vi "Global Aquatrak Output.vi"(0 "AT In":string, 3 "Set Data?":bool) -> (7 "AT Out":string)   [LabVIEW 2018]
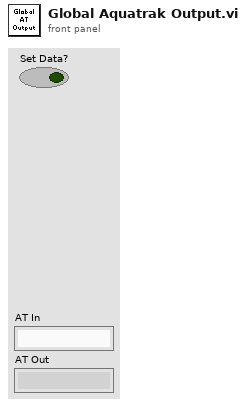
[diagram p1: front panel]
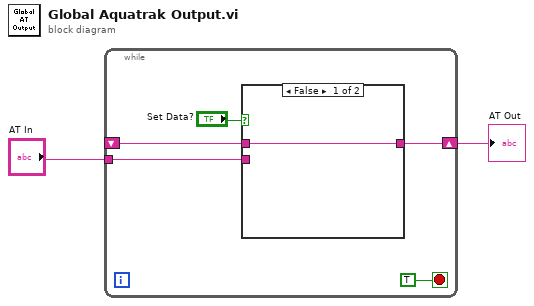
[diagram p0: block diagram]
diagram:
  n1 = while {
    shift-right: [w5] -> w1
    shift-left: _ -> [w4]
    tunnel: "AT In" -> [w3]
    stop <- TRUE stop-if-true
    n2 = case shown="False" "Set Data?" {
      tunnel: [w8 w9] -> w5
      tunnel: w4 -> [w8 _]
      tunnel: w3 -> [_ w9]
      frame False {
      }
      frame True {
      }
    }
  }
  "AT Out" <- w1
